vi "Doppio sensore.vi"() -> ()   [LabVIEW 2021]
uses:
  <vilib>/DAQmx/read.llb/DAQmx Read (Analog 1D Wfm NChan NSamp).vi
  <vilib>/Analysis/baseanly.llb/Mean (DBL).vi
  <vilib>/DAQmx/configure/timing.llb/DAQmx Timing (Sample Clock).vi
  <vilib>/DAQmx/miscellaneous.llb/DAQmx Fill In Error Info.vi
  <vilib>/Utility/file.llb/Write Delimited Spreadsheet (DBL).vi
  <vilib>/Analysis/NI_AALBase.lvlib
panel:
  out "Segnale Proximity 2":dynamicdata(graph)
  in  "File txt Tensione":path
  out "Distanza":dbl[](graph)
  in  "File txt Distanza":path
  out "Media":dbl format="%0.2f"
  out "Deviazione Standard":dbl format="%0.2f"
  out "Massimo":dbl
  out "Minimo":dbl
  in  "STOP":bool
  in  "SAVE":bool
  out "current time":timestamp
  out "Segnale Proximity":dynamicdata(graph)
  out "num campioni":dbl
  in  "Durata":dbl=0.1 format="%.2p"
  in  "Frequenza":dbl=5000.0 format="%0.2p"
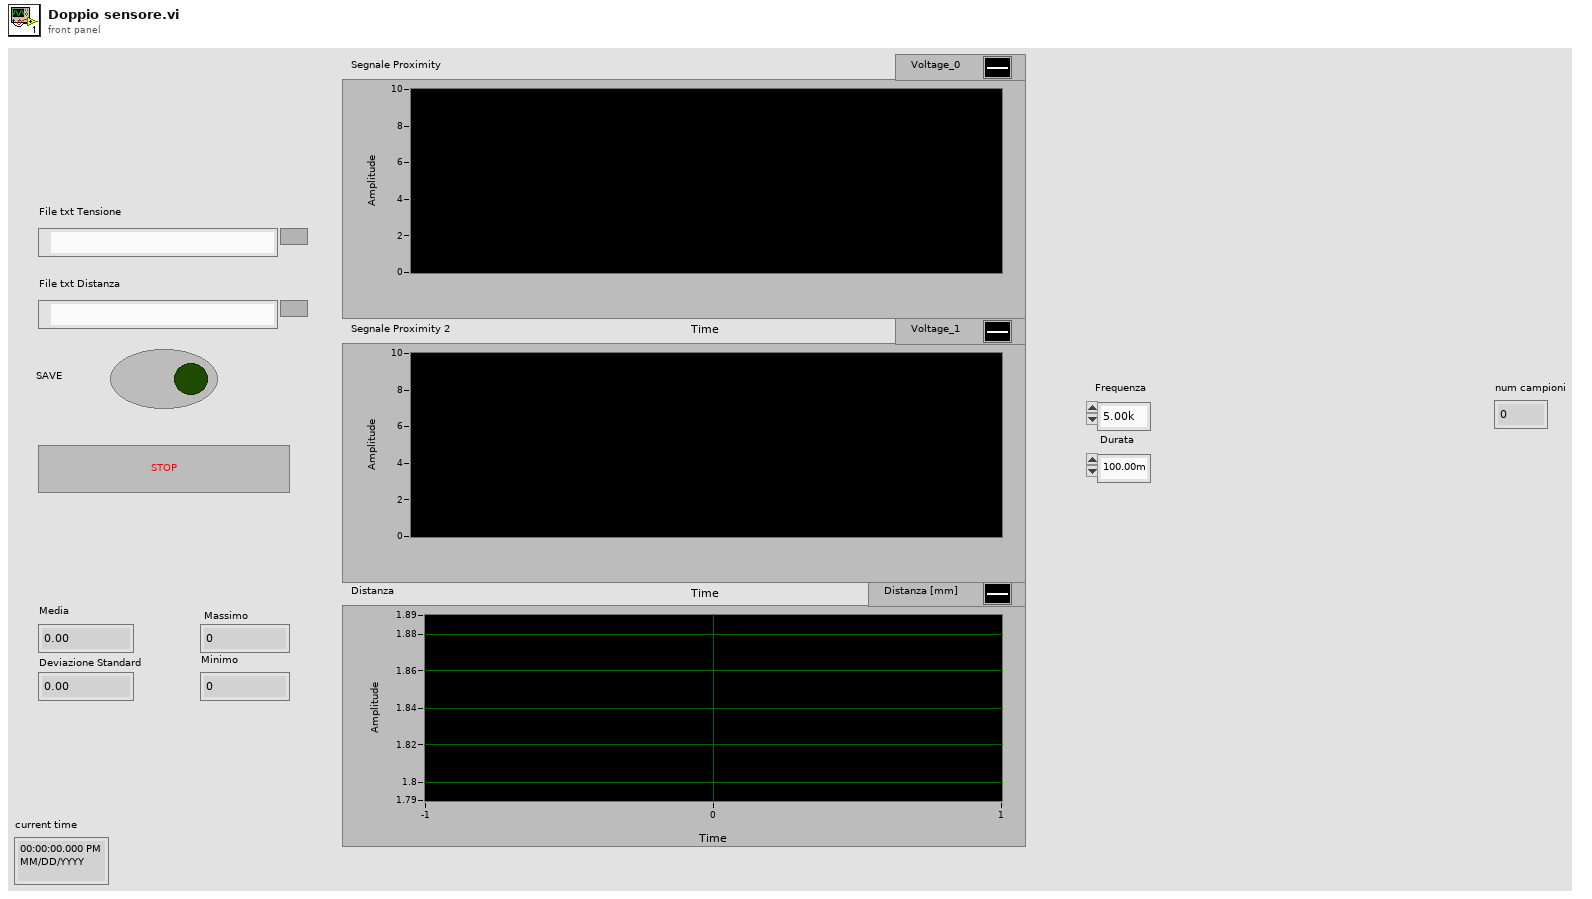
[diagram p1: front panel]
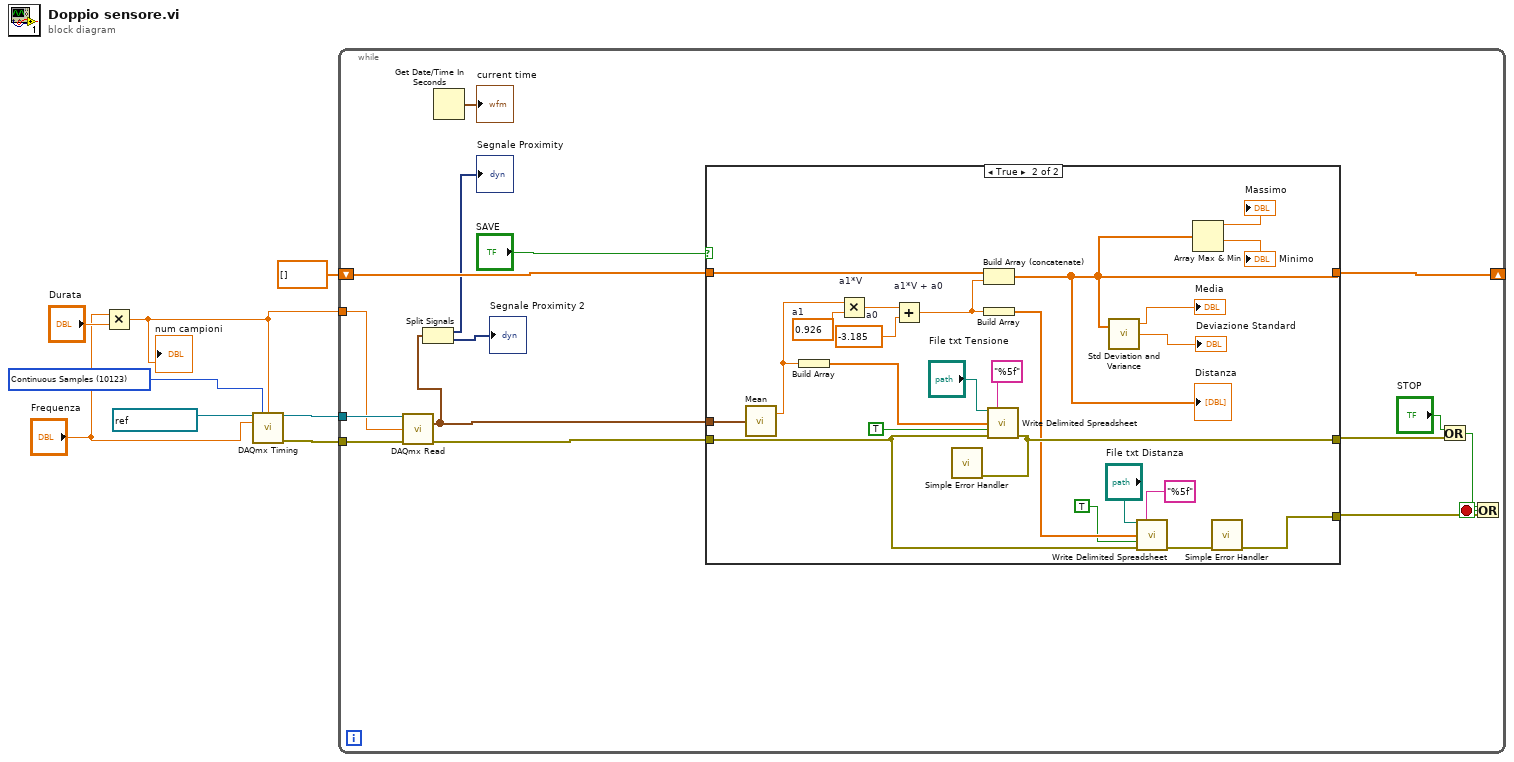
[diagram p0: block diagram]
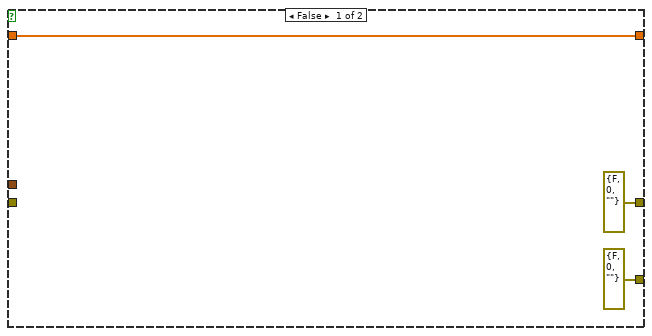
[diagram p2: hidden frame]
diagram:
  w2 = 10123 items=["Finite Samples"=10178, "Continuous Samples"=10123, "Hardware Timed Single Point"=12522] ("sample mode")
  n1 = Multiply(x="Frequenza", y="Durata") -> (x*y=w1:dbl)
  "num campioni" <- w1
  n2 = call-poly <vilib>:"DAQmx Timing.vi"("task/channels in"=refnum<k21> "proximity", "sample mode"=w2, "samples per channel"=w1, "rate"="Frequenza") -> ("task out"=w8:refnum<k21>, "error out"=w5:errorcluster)  [unwired: 10 in]
  n3 = while {
    tunnel: w8 -> [w22]
    tunnel: w1 -> [w12]
    tunnel: w5 -> [w21]
    shift-right: [w17] -> _
    shift-left: dbl[] [] -> [w16]
    stop <- w13 stop-if-true
    n4 = call-poly <vilib>:"DAQmx Read.vi"("task/channels in"=w22, "number of samples per channel"=w12, "error in"=w21) -> ("data"=w11:waveform(dbl)[], "error out"=w19:errorcluster)  [unwired: 10 in, 1 out]
    n5 = Split Signals(w11) -> (→"Segnale Proximity":dynamicdata, →"Segnale Proximity 2":dynamicdata)  [unwired: 2 in]
    n6 = Get Date/Time In Seconds() -> (seconds since 1Jan1904=→"current time":timestamp)
    n7 = case shown="True" "SAVE" {
      tunnel: [errorcluster {"status"=FALSE, "code"=0, "source"=""} ("error IO") w50] -> w23
      tunnel: w11 -> [_ w49]
      tunnel: w19 -> [_ w42]
      tunnel: [w26 w30] -> w17
      tunnel: w16 -> [w26 w33]
      tunnel: [errorcluster {"status"=FALSE, "code"=0, "source"=""} ("error out") w40] -> w15
      frame False {
      }
      frame True {
        w35 = -3.185  # a0
        w36 = 0.926  # a1
        n8 = call-poly <vilib>:"Mean.vi"("X"=w49) -> ("mean"=w37:dbl)  [unwired: 1 out]
        n9 = Build Array(w37) -> (w46:dbl[])
        n10 = Multiply "a1*V"(x=w37, y=w36) -> (x*y=w38:dbl)
        n11 = Add "a1*V + a0"(x=w38, y=w35) -> (x+y=w34:dbl)
        n12 = Build Array (concatenate)(w33, w34) -> (w30:dbl[])
        "Distanza" <- w30
        n13 = Build Array(w34) -> (w45:dbl[])
        n14 = call-poly <vilib>:"Write Delimited Spreadsheet.vi"("file path (dialog if empty)"="File txt Tensione", "format (%.3f)"="%5f", "1D data"=w46, "append to file? (new file:F)"=TRUE, "error in (no error)"=w42) -> ("error out"=w50:errorcluster)  [unwired: 9 in, 1 out]
        n15 = call <vilib>:"Simple Error Handler.vi"("error in (no error)"=w50) -> ()  [unwired: 4 in, 5 out]
        n16 = call <vilib>:"Std Deviation and Variance.vi"("X"=w30) -> ("mean"=→"Media":dbl, "standard deviation"=→"Deviazione Standard":dbl)  [unwired: 1 in, 1 out]
        n17 = call-poly <vilib>:"Write Delimited Spreadsheet.vi"("file path (dialog if empty)"="File txt Distanza", "format (%.3f)"="%5f", "1D data"=w45, "append to file? (new file:F)"=TRUE, "error in (no error)"=w42) -> ("error out"=w41:errorcluster)  [unwired: 9 in, 1 out]
        n18 = Array Max & Min(array=w30) -> (max value=→"Massimo":dbl, min value=→"Minimo":dbl)  [unwired: 2 out]
        n19 = call <vilib>:"Simple Error Handler.vi"("error in (no error)"=w41) -> ("error out"=w40:errorcluster)  [unwired: 4 in, 4 out]
      }
    }
    n20 = Or(x="STOP", y=w23) -> (x .or. y?=w14:bool)
    n21 = Or(x=w14, y=w15) -> (x .or. y?=w13:bool)
  }
